vi "Popup Complex Extended.vi"(8 "error in (no error)":errorcluster, 9 "Panel":refnum<class "Panel.lvclass">, 10 "String in":string, 11 "Numeric Data Type in":refnum<class "Numeric Data Type.lvclass">) -> (0 "error out":errorcluster, 2 "String out":string, 3 "Numeric Data Type out":refnum<class "Numeric Data Type.lvclass">)   [LabVIEW 2018, in "Numeric Data Type.lvclass"]
uses:
  Numeric Data Type.lvclass
  <vilib>/MGI/Panel Manager/Panel/Panel/Panel.lvclass
  Numeric Data Type.lvclass/Numeric Data Type.ctl
  <vilib>/Utility/miscctls.llb/LVPointTypeDef.ctl
  String to Complex Number (CXT).vi
panel:
  in  "Numeric":cxt
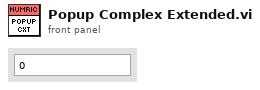
[diagram p1: front panel]
types:
  T1 = typedef "Numeric Data Type.lvclass/Response to Values Outside of Limits Enum.ctl" = enum16{"Ignore", "Coerce to nearest", "Coerce up", "Coerce down"}
  T2 = typedef "LVPointTypeDef.ctl" = cluster{"Horizontal":i16, "Vertical":i16}
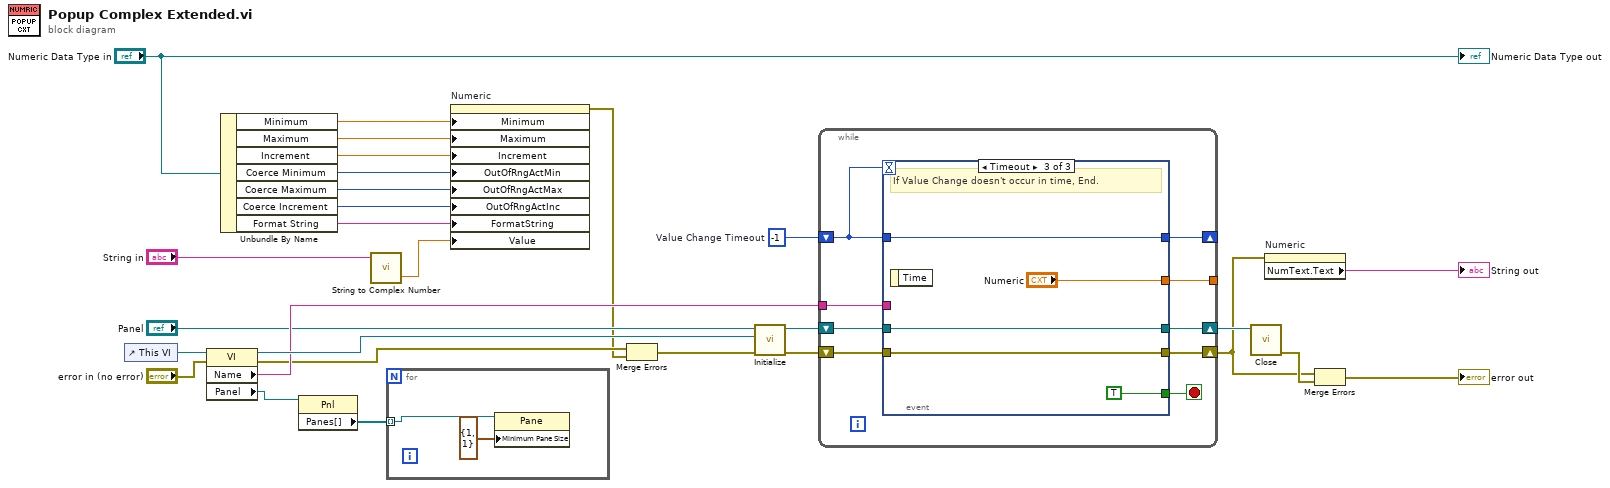
[diagram p0: block diagram]
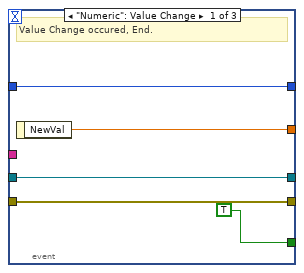
[diagram p2: hidden frame]
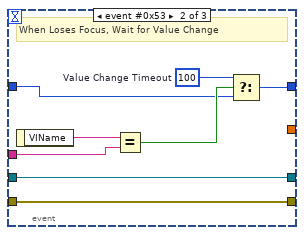
[diagram p3: hidden frame]
diagram:
  w28 = -1  # Value Change Timeout
  n1 = control-ref of="This VI"() -> (w25:refnum<vi>)
  n2 = property class="VI"(reference=w25, error in="error in (no error)") -> (reference out=w24:refnum<vi>, error out=w17:errorcluster, "Name"=w23:string, "Panel"=w6:refnum<vi>)
  n3 = Unbundle By Name("Numeric Data Type in") -> ("Minimum"=w16:dbl, "Maximum"=w15:dbl, "Increment"=w14:dbl, "Coerce Minimum"=w13:T1, "Coerce Maximum"=w12:T1, "Coerce Increment"=w11:T1, "Format String"=w10:string)
  n4 = property class="Pnl"(reference=w6) -> ("Panes[]"=w5:refnum<vi>[])  [unwired: 1 in, 2 out]
  n5 = call-poly "String to Complex Number.vi"("string"="String in") -> ("number"=w3:cxt)  [unwired: 3 in, 1 out]
  n6 = for {
    tunnel: w5 -> [w30] mode=indexing
    n7 = property class="Pane"(reference=w30, "Minimum Pane Size"=T2 {"Horizontal"=1, "Vertical"=1}) -> ()  [unwired: 1 in, 2 out]
  }
  n8 = property on="Numeric" class="DigNum (strict)"("Minimum"=w16, "Maximum"=w15, "Increment"=w14, "OutOfRngActMin"=w13, "OutOfRngActMax"=w12, "OutOfRngActInc"=w11, "FormatString"=w10, "Value"=w3) -> (error out=w8:errorcluster)  [unwired: 2 in, 1 out]
  n9 = Merge Errors(w17, w8) -> (w9:errorcluster)
  n10 = call <vilib>:"Initialize.vi"("error in (no error)"=w9, "VI Refnum"=w24, "Panel In"="Panel") -> ("error out"=w26:errorcluster, "Panel Out"=w27:refnum<class "Panel.lvclass">)  [unwired: 6 in, 1 out]
  n11 = while {
    shift-right: [w39] -> w2
    shift-left: w26 -> [w38]
    shift-right: [w36] -> w21
    shift-left: w27 -> [w35]
    tunnel: [w34] -> _
    tunnel: w23 -> [w33]
    shift-right: [w31] -> _
    shift-left: w28 -> [w32]
    stop <- w37 stop-if-true
    n12 = event shown="[2] Timeout" {
      selector: _ -> [_ _ _]
      dyn-events: _ -> [_ _ _]
      timeout: w32 -> [_ _ _]
      tunnel: [w41 w50 w55] -> w39
      tunnel: w38 -> [w41 w50 w55]
      tunnel: [TRUE _ TRUE] -> w37
      tunnel: [w43 w49 w56] -> w36
      tunnel: w35 -> [w43 w49 w56]
      tunnel: [w42 _ "Numeric"] -> w34
      tunnel: w33 -> [_ w51 _]
      tunnel: w32 -> [w40 w46 w53]
      tunnel: [w40 w45 w53] -> w31
      event "Numeric": Value Change {
        # "Value Change occured, End."
        n13 = event-data() -> ("NewVal"=w42:cxt)  [unwired: 1 in]
      }
      event event #0x53 {
        w47 = 100  # Value Change Timeout
        # "When Loses Focus, Wait for Value Change"
        n14 = event-data() -> ("VIName"=w52:string)  [unwired: 1 in]
        n15 = Equal?(x=w52, y=w51) -> (x = y?=w48:bool)
        n16 = Select(t=w47, s=w48, f=w46) -> (s? t:f=w45:i32)
      }
      event Timeout {
        # "If Value Change doesn't occur in time, End."
        n17 = event-data() -> ()  [unwired: 1 in, 1 out]
      }
    }
  }
  n18 = call-dynamic "Close.vi"("Panel In"=w21) -> ("Error Out"=w22:errorcluster)  [unwired: 10 in]
  n19 = property on="Numeric" class="DigNum (strict)"(error in=w2) -> ("NumText.Text"=→"String out":string)  [unwired: 1 in, 2 out]
  n20 = Merge Errors(w2, w22) -> (→"error out":errorcluster)
  "Numeric Data Type out" <- "Numeric Data Type in"
